vi "test-datamemberaccess.vi"() -> ()   [LabVIEW 2026]
doc: "<b>Code Developed By:</b> +\nDaniel Coons +\nTechnology Service Corporation +\nwww.tsc.com/atcs"
uses:
  Material-Scheme.lvclass
  data member access/get surfaceBright.vi
  data member access/Get onError.vi
panel:
  out "concatenated string":string
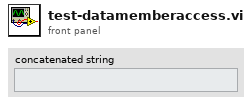
[diagram p1: front panel]
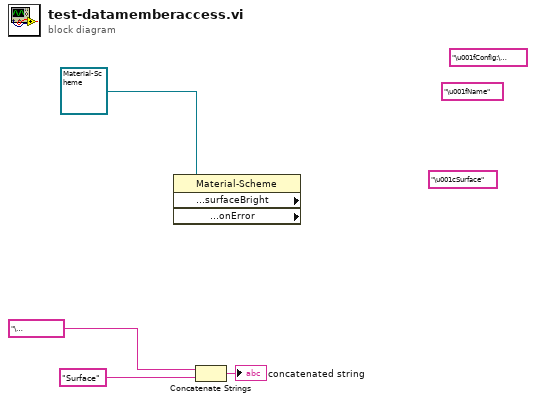
[diagram p0: block diagram]
diagram:
  (unwired) "\u001fName"
  (unwired) "\u001cSurface"
  (unwired) "\u001fConfig:\u001fN"
  n1 = property class="Material-Scheme" props=["data member access:Surface:surfaceBright", "data member access:Text Colors:onError"](reference=refnum<class "Material-Scheme.lvclass"> refnum ("TSC Material Theme.lvlib:Material-Scheme")) -> ()  [unwired: 1 in, 4 out]
  n2 = Concatenate Strings("\u0000Surface", "Surface" ("string")) -> (→"concatenated string":string)
